vi "Konvolucio MUDS150628 B232EATC Session Read DTC TesterPresent.vi"() -> ()   [LabVIEW 2011]
uses:
  <instrlib>/Konvolucio MUDS150628/Types/DtcItemType.ctl
  <instrlib>/Konvolucio MUDS150628/Konvolucio MUDS150628.lvlib
panel:
  out "DtcItems":T1[](array[typedef])
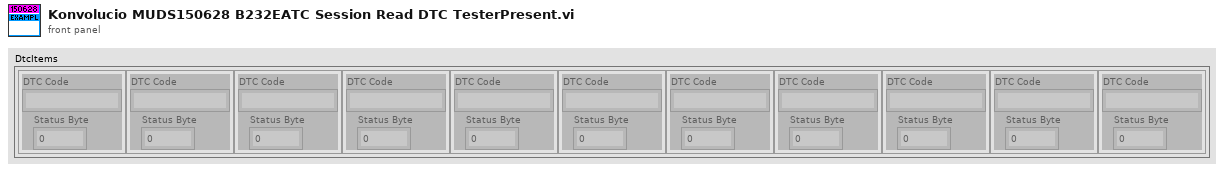
[diagram p1: front panel]
types:
  T1 = typedef "Konvolucio MUDS150628.lvlib/DtcItemType.ctl" = cluster{"DTC Code":string, "Status Byte":i32}
  T2 = typedef "Konvolucio MUDS150628.lvlib/UdsHandleType.ctl" = cluster{"LogPath":path, "LogEnabled":bool, "isOpen":bool, "LogContent":string, "Adapter":string, "MCanHandle":T3, "TransmittId":u32, "ReceiveId":u32}
  T3 = typedef "Konvolucio MCAN120803.lvlib/MCanHandleType.ctl" = cluster{"MCanAdapter":refnum<k24>}
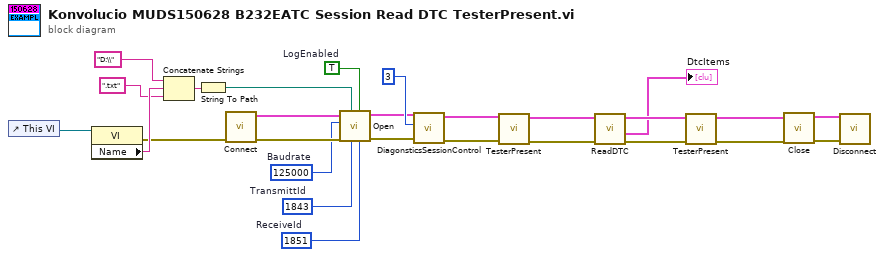
[diagram p0: block diagram]
diagram:
  w9 = TRUE  # LogEnabled
  w8 = u32 125000  # Baudrate
  w5 = u32 1851  # ReceiveId
  w6 = u32 1843  # TransmittId
  n1 = control-ref of="This VI"() -> (w17:refnum<vi>)
  n2 = property class="VI"(reference=w17) -> (error out=w12:errorcluster, "Name"=w15:string)  [unwired: 1 in, 1 out]
  n3 = Concatenate Strings("D:\\" ("VI Name"), w15, ".txt" ("string")) -> (w13:string)
  n4 = String To Path(string=w13) -> (path=w7:path)
  n5 = call <instrlib>:"Connect.vi"("error in"=w12) -> ("error out"=w10:errorcluster, "UdsHandleOut"=w11:T2)  [unwired: 9 in]
  n6 = call <instrlib>:"Open.vi"("ReceiveId"=w5, "LogEnabled"=w9, "TransmittId"=w6, "LogPath"=w7, "error in"=w10, "BaudRate"=w8, "UdsHandleIn"=w11) -> ("error out"=w4:errorcluster, "UdsHandleOut"=w3:T2)  [unwired: 3 in]
  n7 = call <instrlib>:"DiagonsticsSessionControl.vi"("error in"=w4, "Session"=u8 3, "UdsHandleIn"=w3) -> ("error out"=w25:errorcluster, "UdsHandleOut"=w24:T2)  [unwired: 7 in]
  n8 = call <instrlib>:"TesterPresent.vi"("error in"=w25, "UdsHandleIn"=w24) -> ("error out"=w22:errorcluster, "UdsHandleOut"=w21:T2)  [unwired: 8 in]
  n9 = call <instrlib>:"ReadDTC.vi"("error in"=w22, "UdsHandleIn"=w21) -> ("error out"=w20:errorcluster, "DtcItems"=→"DtcItems":T1[], "UdsHandleOut"=w19:T2)  [unwired: 6 in, 1 out]
  n10 = call <instrlib>:"TesterPresent.vi"("error in"=w20, "UdsHandleIn"=w19) -> ("error out"=w27:errorcluster, "UdsHandleOut"=w26:T2)  [unwired: 8 in]
  n11 = call <instrlib>:"Close.vi"("error in"=w27, "UdsHandleIn"=w26) -> ("error out"=w2:errorcluster, "UdsHandleOut"=w1:T2)  [unwired: 8 in]
  n12 = call <instrlib>:"Disconnect.vi"("error in"=w2, "UdsHandleIn"=w1) -> ()  [unwired: 9 in, 1 out]
